vi "_Start Animation.vi"(8 "Error In":errorcluster, 11 "Animation Config":T1) -> (0 "Error Out":errorcluster, 3 "Animation Config":T1)   [LabVIEW 2011, in "LVH-Build-Tools.lvlib"]
uses:
  LVH-Build-Tools.lvlib
  _Animation Config.ctl
  <vilib>/picture/picture.llb/imagedata.ctl
  _Animation FGV State.ctl
panel:
  in  "Error In 2":errorcluster
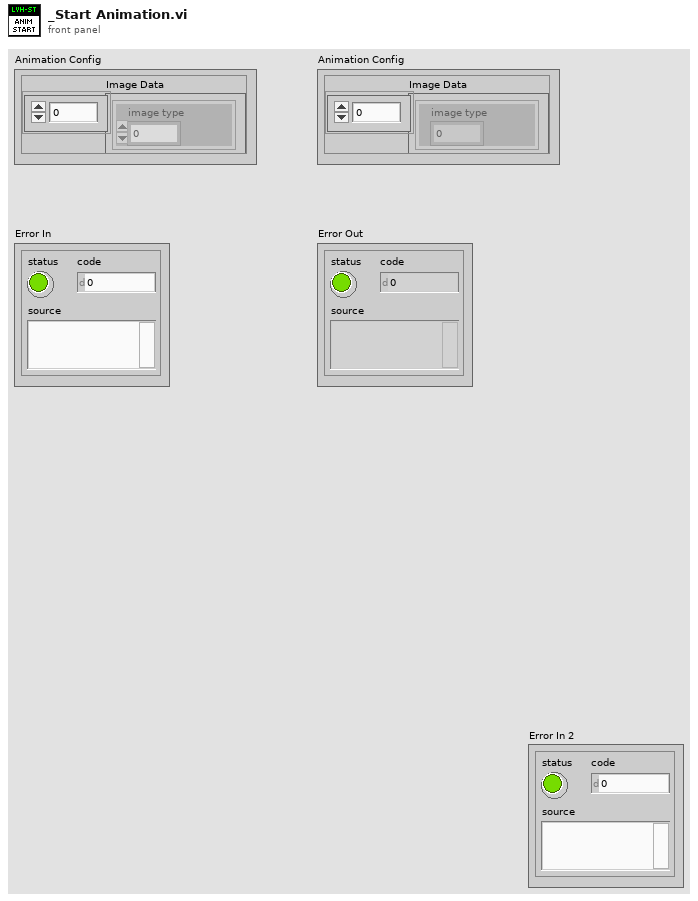
[diagram p1: front panel]
types:
  T1 = typedef "LVH-Build-Tools.lvlib/_Animation Config.ctl" = cluster{"Image Data":T2[], "Animation Picture Indicator":refnum<vi>, "FPS":u32, "Position":cluster{"X":i16, "Y":i16}}
  T2 = typedef "imagedata.ctl" = cluster{"image type":i32, "image depth":i32, "image":u8[], "mask":u8[], "colors":u32[], "Rectangle":cluster{"left":i16, "top":i16, "right":i16, "bottom":i16}}
  T3 = enum32{"invalid app kind", "Development System", "Run Time System", "Student Edition", "Embedded LabVIEW", "Evaluation", "Custom"}
  T4 = typedef "LVH-Build-Tools.lvlib/_Animation FGV State.ctl" = enum16{"Init", "Set", "Get"}
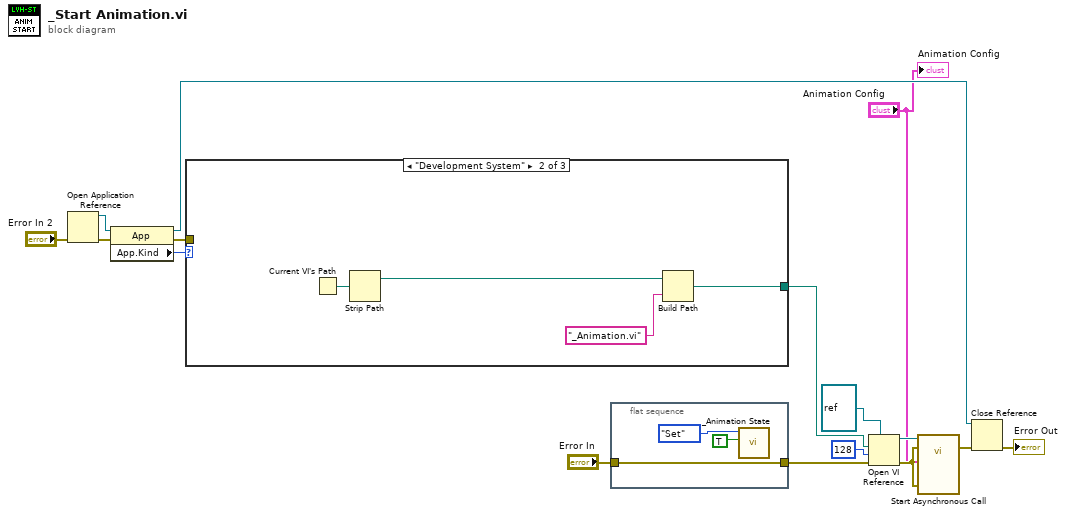
[diagram p0: block diagram]
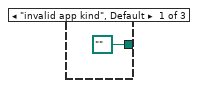
[diagram p2: hidden frame]
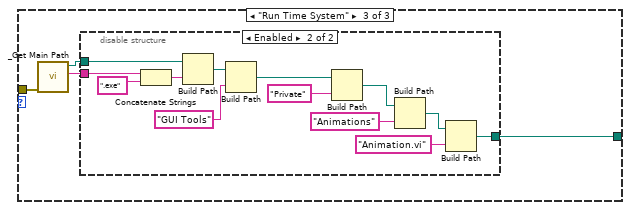
[diagram p3: hidden frame]
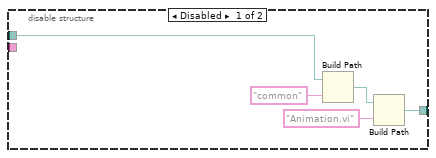
[diagram p4: hidden frame]
diagram:
  n1 = Open Application Reference(8:"Error In 2") -> (0:w11:errorcluster, 3:w10:refnum<vi>)  [unwired: 3 in]
  n2 = property class="App"(reference=w10, error in=w11) -> (reference out=w5:refnum<vi>, error out=w7:errorcluster, "App.Kind"=w9:T3)
  n3 = case shown="\"Development System\"" w9 {
    tunnel: [path "" ("appended path") w19 w23] -> w8
    tunnel: w7 -> [_ _ w24]
    frame "invalid app kind", Default {
    }
    frame "Development System" {
      n4 = Current VI's Path() -> (path=w21:path)
      n5 = Strip Path(path=w21) -> (stripped path=w18:path)  [unwired: 1 out]
      n6 = Build Path(base path=w18, name or relative path="_Animation.vi") -> (appended path=w19:path)
    }
    frame "Run Time System" {
      n7 = call "_Get Main Path.vi"("Error In"=w24) -> ("Main Name"=w22:string, "Main Dir"=w25:path)  [unwired: 8 in, 1 out]
      n8 = disable-structure shown="Enabled" {
        disable-tunnel: w25 -> [w30 w35]
        disable-tunnel: [w26 w39] -> w23
        disable-tunnel: w22 -> [_ w33]
        frame Disabled {
          n9 = Build Path(base path=w30, name or relative path="common") -> (appended path=w27:path)
          n10 = Build Path(base path=w27, name or relative path="Animation.vi") -> (appended path=w26:path)
        }
        frame Enabled {
          n11 = Concatenate Strings(w33, ".exe" ("string")) -> (w32:string)
          n12 = Build Path(base path=w35, name or relative path=w32) -> (appended path=w36:path)
          n13 = Build Path(base path=w36, name or relative path="GUI Tools") -> (appended path=w38:path)
          n14 = Build Path(base path=w38, name or relative path="Private") -> (appended path=w31:path)
          n15 = Build Path(base path=w31, name or relative path="Animations") -> (appended path=w37:path)
          n16 = Build Path(base path=w37, name or relative path="Animation.vi") -> (appended path=w39:path)
        }
      }
    }
  }
  n17 = flat-sequence {
    tunnel: [w44] -> w14
    tunnel: "Error In" -> [w44]
    frame #0 {
      n18 = call "_Animation State.vi"("Running?"=TRUE, "Function"=_Animation_FGV_State."Set") -> ()  [unwired: 9 in, 1 out]
    }
  }
  n19 = Open VI Reference(type specifier VI Refnum (for type only)=refnum<vi> refnum, vi path=w8, options=128, error in (no error)=w14) -> (vi reference=w4:refnum<vi>, error out=w3:errorcluster)  [unwired: 2 in]
  n20 = call-by-ref "Start Asynchronous Call"(reference=w4, error in=w3, "Error In"=w3, "Animation Config"="Animation Config") -> (error out=w2:errorcluster)  [unwired: 8 in, 3 out]
  n21 = Close Reference(reference=w5, error in (no error)=w2) -> (error out=→"Error Out":errorcluster)
  "Animation Config" <- "Animation Config"
